vi "TDC_enableTdcInput.vi"(8 "Error In":errorcluster, 11 "Enable":bool) -> (0 "Error Out":errorcluster)   [LabVIEW 2011]
uses:
  tdcbase.dll
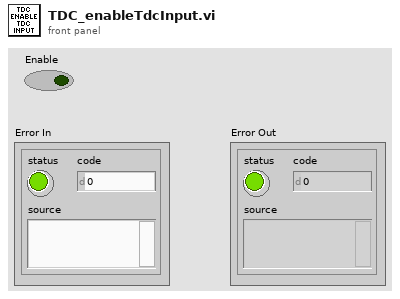
[diagram p1: front panel]
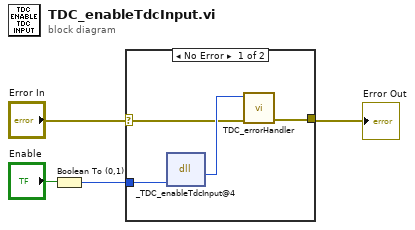
[diagram p0: block diagram]
diagram:
  n1 = Boolean To (0,1)(Boolean="Enable") -> (0, 1=w2:i16)
  n2 = case shown="No Error" "Error In" {
    selector: "Error In" -> [w5 w9]
    tunnel: [w7 w9] -> w4
    tunnel: w2 -> [w6 _]
    frame No Error {
      n3 = dll-call lib="X:/tdcbase.dll" fn="_TDC_enableTdcInput@4"("enable"=w6) -> ("return type"=w8:i32)  [unwired: 4 in, 2 out]
      n4 = call "TDC_errorHandler.vi"("Error In"=w5, "TDC Return Code"=w8) -> ("Error Out"=w7:errorcluster)  [unwired: 9 in]
    }
    frame Error {
    }
  }
  "Error Out" <- w4
